vi "Simple Dual Mode Thermometer Facade.vi"(9 "Container State":T3, 10 "Display State In":T2, 11 "Data In":T4) -> (0 "Action":T1, 1 "Display State Out":T2, 3 "Data Out":T4)   [LabVIEW 2023, in "Simple Dual Mode Thermometer XControl.xctl"]
doc: "This VI demonstrates the use of an XControl's Facade VI in implementing a Simple Dual Mode Thermometer. The front panel defines the appearance of the XControl. The block diagram defines the behavior of the XControl."
uses:
  Simple Dual Mode Thermometer XControl.xctl
  Simple Dual Mode Thermometer Data.ctl
  <vilib>/_xctls/Container State.ctl
  Simple Dual Mode Thermometer State.ctl
  <vilib>/_xctls/Action.ctl
  <vilib>/_xctls/XControlSupport.lvlib
panel:
  in  "format string":string="The temperature is %f degrees C or %f degrees F."
  in  "Item Name":string="Display Temperature..."
  in  "Action Name":string="Mode Change"
  in  "Fahrenheit":bool
  in  "Vertical Pointer Slide":dbl(slide) scale=0.0..100.0
  in  "Thermometer":dbl(slide) scale=0.0..100.0
  # "1. Drop the controls that make up the appearance of the XControl here.\n2. Resize the window to fit the controls.\n3. If the XControl is of fixed size,  make the window not resizable from VI Properties->Window Appearance.\n4. If you want the controls to automatically size when the XControl sizes, check  \"Scale all objects on front panel when window resizes\" in File->VI Properties->Window Size page."
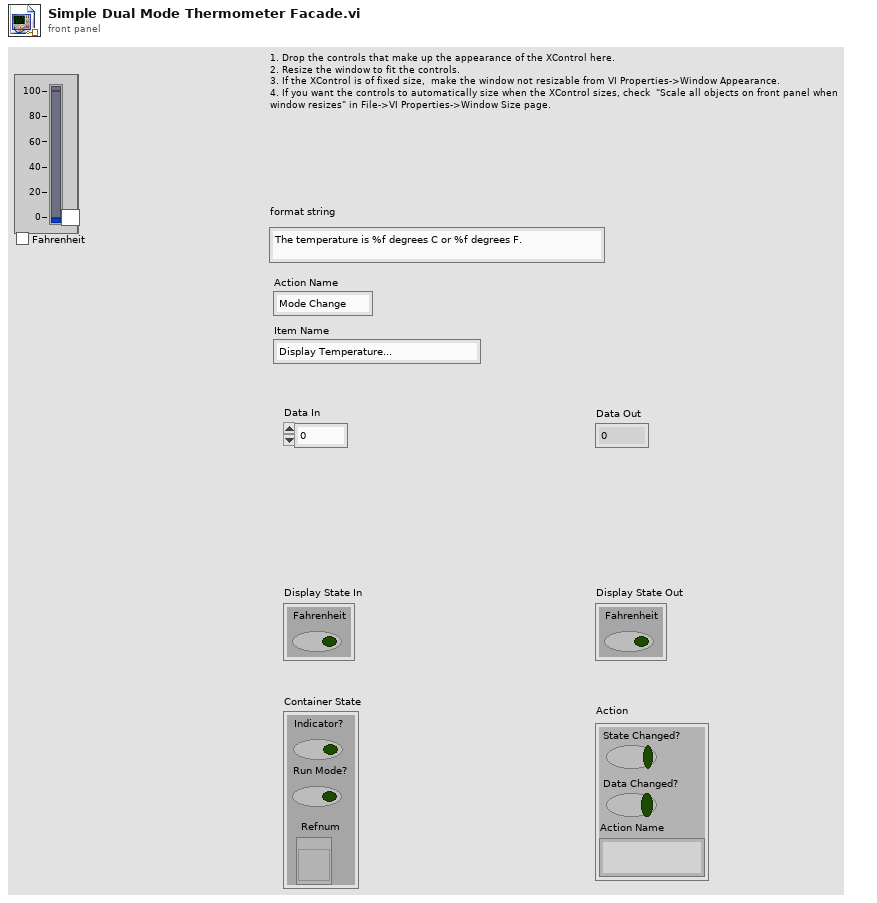
[diagram p1: front panel]
types:
  T1 = typedef "XControlSupport.lvlib/Action.ctl" = cluster{"Data Changed?":bool, "State Changed?":bool, "Action Name":string}
  T2 = typedef "Simple Dual Mode Thermometer XControl.xctl/Simple Dual Mode Thermometer State.ctl" = cluster{"Fahrenheit":bool}
  T3 = typedef "XControlSupport.lvlib/Container State.ctl" = cluster{"Indicator?":bool, "Run Mode?":bool, " Refnum":refnum<vi>}
  T4 = typedef "Simple Dual Mode Thermometer XControl.xctl/Simple Dual Mode Thermometer Data.ctl" = dbl
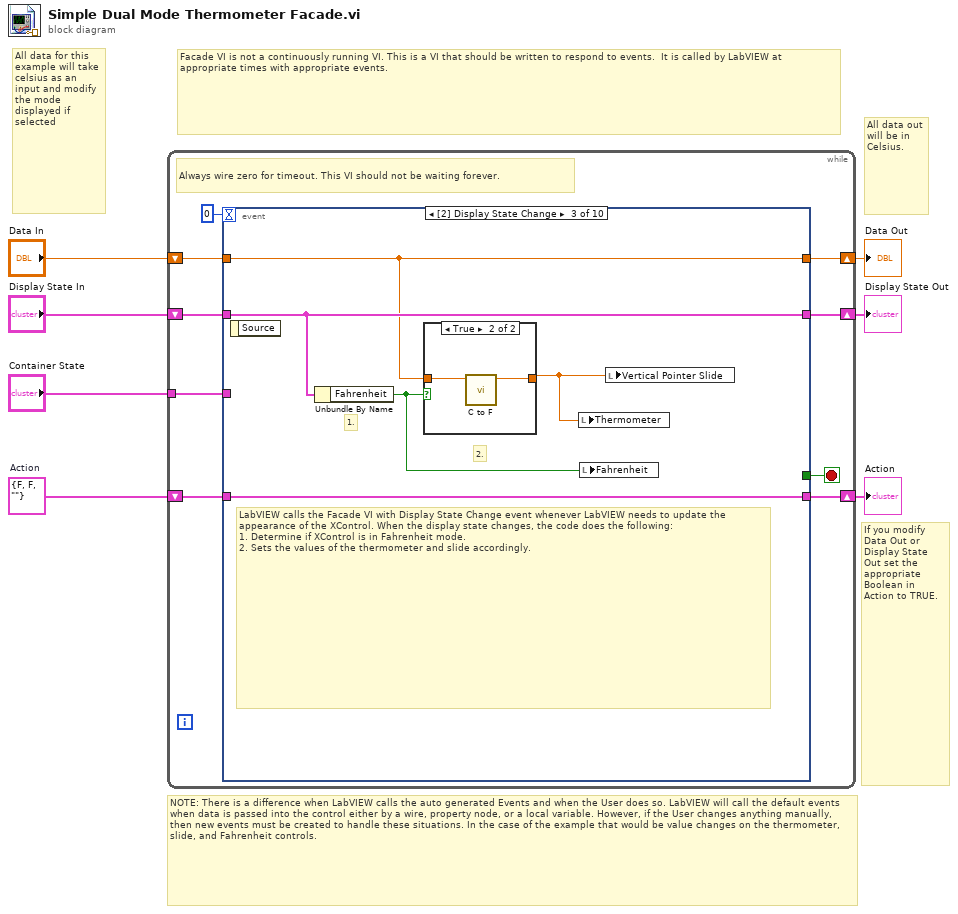
[diagram p0: block diagram]
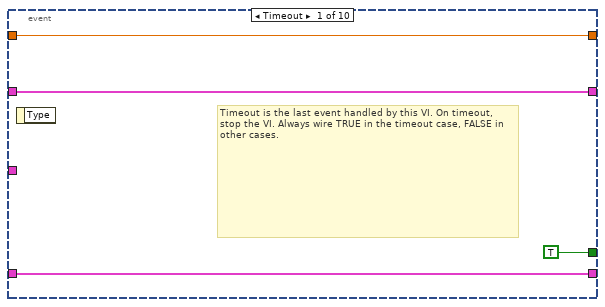
[diagram p2: hidden frame]
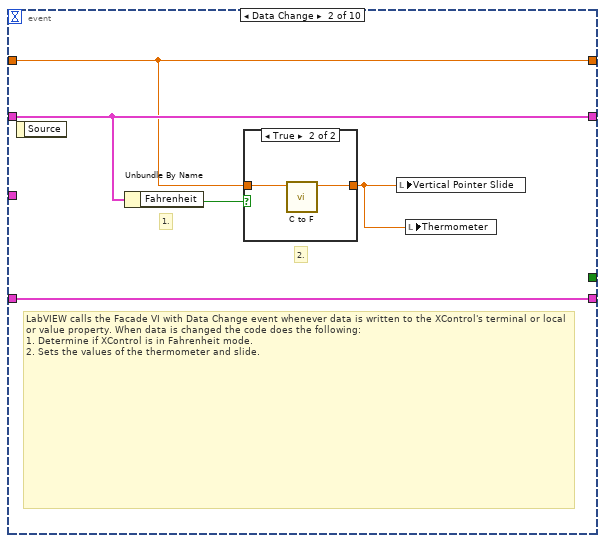
[diagram p3: hidden frame]
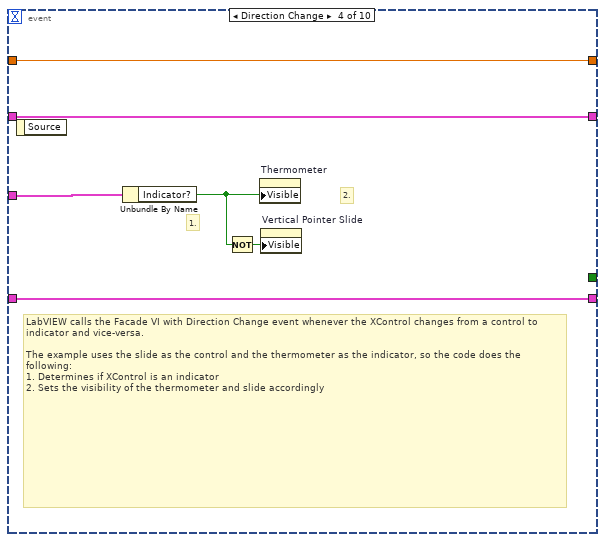
[diagram p6: hidden frame]
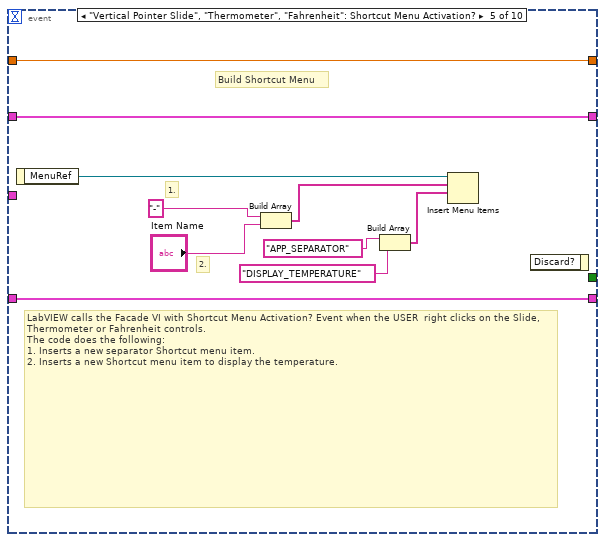
[diagram p7: hidden frame]
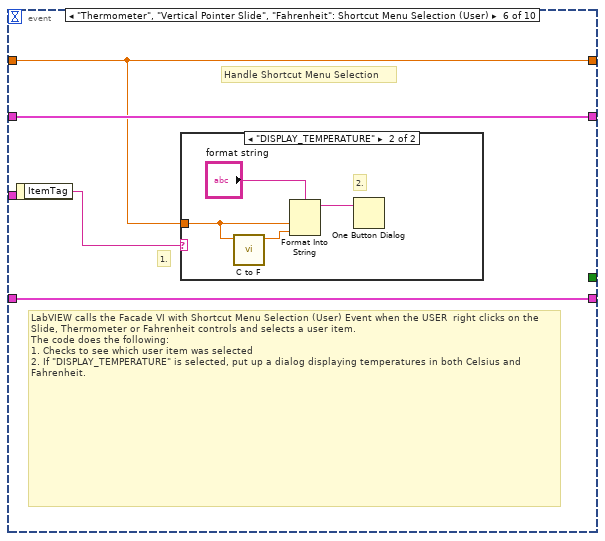
[diagram p8: hidden frame]
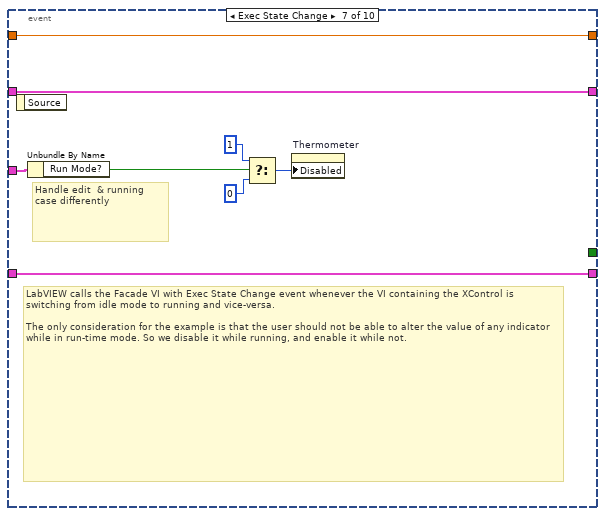
[diagram p10: hidden frame]
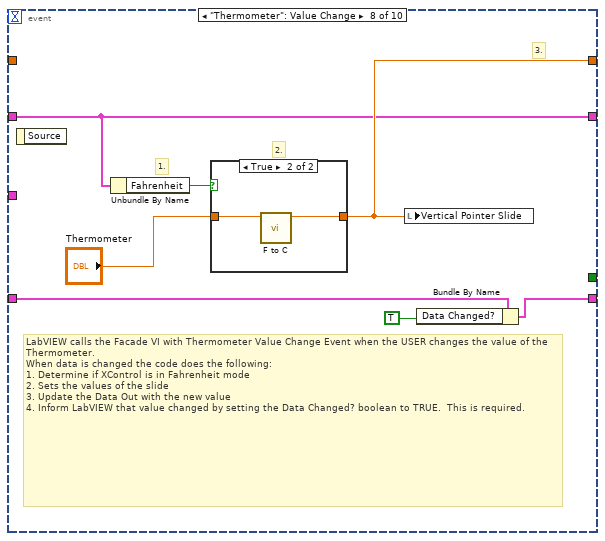
[diagram p11: hidden frame]
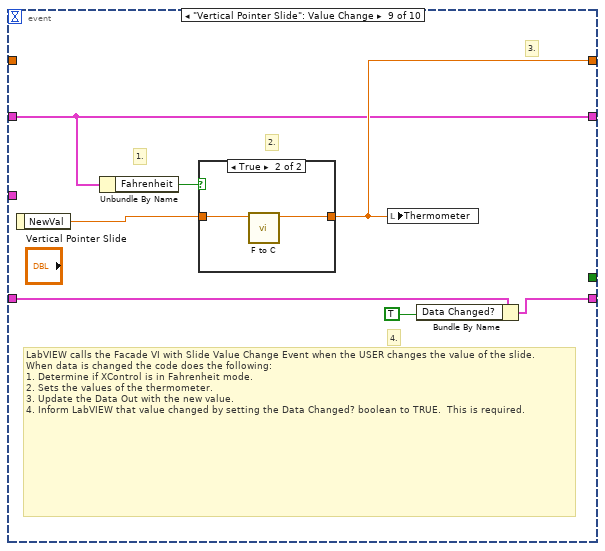
[diagram p13: hidden frame]
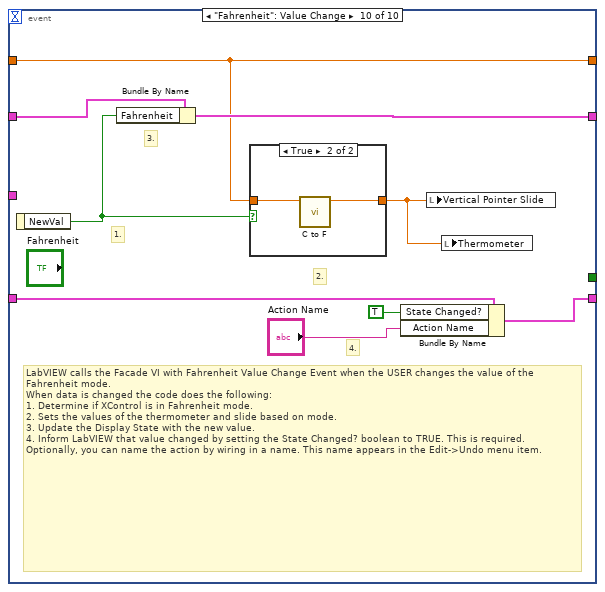
[diagram p15: hidden frame]
diagram:
  w1 = T1 {"Data Changed?"=FALSE, "State Changed?"=FALSE, "Action Name"=""}  # Action
  # "Facade VI is not a continuously running VI. This is a VI that should be written to respond to events.  It is called by LabVIEW at appropriate times with appropriate events."
  # "NOTE: There is a difference when LabVIEW calls the auto generated Events and when the User does so. LabVIEW will call the default events when data is passed into the control either by a wire, property node, or a local variable. However, if the User changes anything manually, then new events must be created to handle these situations. In the case of the example that would be value changes on the thermometer, slide, and Fahrenheit controls."
  # "All data out will be in Celsius."
  # "All data for this example will take celsius as an input and modify the mode displayed if selected"
  # "If you modify Data Out or\nDisplay State Out set the appropriate Boolean in Action to TRUE."
  n1 = while {
    shift-right: [w15] -> w4
    shift-left: "Display State In" -> [w16]
    tunnel: "Container State" -> [w12]
    shift-right: [w10] -> w7
    shift-left: "Data In" -> [w11]
    shift-right: [w8] -> w2
    shift-left: w1 -> [w9]
    stop <- w14 stop-if-true
    # "Always wire zero for timeout. This VI should not be waiting forever."
    n2 = event shown="[2] Display State Change" {
      selector: _ -> [_ _ _ _ _ _ _ _ _ _]
      dyn-events: _ -> [_ _ _ _ _ _ _ _ _ _]
      timeout: 0 -> [_ _ _ _ _ _ _ _ _ _]
      tunnel: w16 -> [w18 w25 w33 w41 w50 w55 w67 w71 w80 w97]
      tunnel: [w18 w25 w33 w41 w50 w55 w67 w71 w80 w96] -> w15
      tunnel: [TRUE _ _ _ _ _ _ _ _ _] -> w14
      tunnel: w12 -> [_ _ _ w42 _ _ w68 _ _ _]
      tunnel: w11 -> [w17 w23 w32 w40 w51 w53 w66 _ _ w95]
      tunnel: [w17 w23 w32 w40 w51 w53 w66 w72 w81 w95] -> w10
      tunnel: [w19 w21 w30 w37 w52 w56 w65 w73 w82 w91] -> w8
      tunnel: w9 -> [w19 w21 w30 w37 w52 w56 w65 w74 w83 w94]
      event Timeout {
        # "Timeout is the last event handled by this VI. On timeout, stop the VI. Always wire TRUE in the timeout case, FALSE in other cases."
        n3 = event-data() -> ()  [unwired: 1 in, 1 out]
      }
      event Data Change {
        # "2."
        # "1."
        # "LabVIEW calls the Facade VI with Data Change event whenever data is written to the XControl's terminal or local or value property. When data is changed the code does the following:\n1. Determine if XControl is in Fahrenheit mode.\n2. Sets the values of the thermometer and slide."
        n4 = event-data() -> ()  [unwired: 1 in, 1 out]
        n5 = Unbundle By Name(w25) -> ("Fahrenheit"=w24:bool)
        n6 = case shown="True" w24 {
          tunnel: w23 -> [w26 w28]
          tunnel: [w26 w27] -> w22
          frame False {
          }
          frame True {
            n7 = call "C to F.vi"("Celsius"=w28) -> ("Fahrenheit"=w27:dbl)  [unwired: 10 in]
          }
        }
        n8 = local write "Vertical Pointer Slide"(w22) -> ()
        n9 = local write "Thermometer"(w22) -> ()
      }
      event Display State Change {
        # "2."
        # "1."
        # "LabVIEW calls the Facade VI with Display State Change event whenever LabVIEW needs to update the appearance of the XControl. When the display state changes, the code does the following:\n1. Determine if XControl is in Fahrenheit mode.\n2. Sets the values of the thermometer and slide accordingly."
        n10 = event-data() -> ()  [unwired: 1 in, 1 out]
        n11 = Unbundle By Name(w33) -> ("Fahrenheit"=w29:bool)
        n12 = case shown="True" w29 {
          tunnel: w32 -> [w34 w36]
          tunnel: [w34 w35] -> w31
          frame False {
          }
          frame True {
            n13 = call "C to F.vi"("Celsius"=w36) -> ("Fahrenheit"=w35:dbl)  [unwired: 10 in]
          }
        }
        n14 = local write "Thermometer"(w31) -> ()
        n15 = local write "Fahrenheit"(w29) -> ()
        n16 = local write "Vertical Pointer Slide"(w31) -> ()
      }
      event Direction Change {
        # "2."
        # "1."
        # "LabVIEW calls the Facade VI with Direction Change event whenever the XControl changes from a control to indicator and vice-versa.\n\nThe example uses the slide as the control and the thermometer as the indicator, so the code does the following: \n1. Determines if XControl is an indicator \n2. Sets the visibility of the thermometer and slide accordingly"
        n17 = event-data() -> ()  [unwired: 1 in, 1 out]
        n18 = Unbundle By Name(w42) -> ("Indicator?"=w38:bool)
        n19 = Not(x=w38) -> (.not. x?=w39:bool)
        n20 = property on="Thermometer" class="Slide (strict)"("Visible"=w38) -> ()  [unwired: 2 in, 2 out]
        n21 = property on="Vertical Pointer Slide" class="Slide (strict)"("Visible"=w39) -> ()  [unwired: 2 in, 2 out]
      }
      event "Vertical Pointer Slide", "Thermometer", "Fahrenheit": Shortcut Menu Activation? {
        # "Build Shortcut Menu"
        # "2."
        # "1."
        # "LabVIEW calls the Facade VI with Shortcut Menu Activation? Event when the USER  right clicks on the Slide, Thermometer or Fahrenheit controls.\nThe code does the following:\n1. Inserts a new separator Shortcut menu item.\n2. Inserts a new Shortcut menu item to display the temperature."
        n22 = event-data() -> ("MenuRef"=w46:refnum<k9>)  [unwired: 1 in]
        n23 = Build Array("-", "Item Name") -> (w47:string[])
        n24 = Build Array("APP_SEPARATOR", "DISPLAY_TEMPERATURE" ("element")) -> (w45:string[])
        n25 = Insert Menu Items(7:w45, 8:w47, 9:w46) -> ()  [unwired: 3 in, 3 out]
        n26 = event-data() -> ()  [unwired: 2 in, 1 out]
      }
      event "Thermometer", "Vertical Pointer Slide", "Fahrenheit": Shortcut Menu Selection (User) {
        # "Handle Shortcut Menu Selection"
        # "1."
        # "LabVIEW calls the Facade VI with Shortcut Menu Selection (User) Event when the USER  right clicks on the Slide, Thermometer or Fahrenheit controls and selects a user item.\nThe code does the following:\n1. Checks to see which user item was selected\n2. If \"DISPLAY_TEMPERATURE\" is selected, put up a dialog displaying temperatures in both Celsius and Fahrenheit."
        n27 = event-data() -> ("ItemTag"=w54:string)  [unwired: 1 in]
        n28 = case shown="\"DISPLAY_TEMPERATURE\"" w54 {
          tunnel: w53 -> [_ w57]
          frame Default {
          }
          frame "DISPLAY_TEMPERATURE" {
            # "2."
            n29 = call "C to F.vi"("Celsius"=w57) -> ("Fahrenheit"=w58:dbl)  [unwired: 10 in]
            n30 = Format Into String(format string="format string", w57, w58) -> (resulting string=w59:string)  [unwired: 2 in, 1 out]
            n31 = One Button Dialog(message=w59) -> ()  [unwired: 1 in, 1 out]
          }
        }
      }
      event Exec State Change {
        # "LabVIEW calls the Facade VI with Exec State Change event whenever the VI containing the XControl is switching from idle mode to running and vice-versa.\n\nThe only consideration for the example is that the user should not be able to alter the value of any indicator while in run-time mode. So we disable it while running, and enable it while not."
        # "Handle edit  & running case differently"
        n32 = event-data() -> ()  [unwired: 1 in, 1 out]
        n33 = Unbundle By Name(w68) -> ("Run Mode?"=w64:bool)
        n34 = Select(t=u8 1 ("Disabled"), s=w64, f=u8 0 ("Disabled")) -> (s? t:f=w61:u8)
        n35 = property on="Thermometer" class="Slide (strict)"("Disabled"=w61) -> ()  [unwired: 2 in, 2 out]
      }
      event "Thermometer": Value Change {
        # "LabVIEW calls the Facade VI with Thermometer Value Change Event when the USER changes the value of the Thermometer.\nWhen data is changed the code does the following:\n1. Determine if XControl is in Fahrenheit mode\n2. Sets the values of the slide\n3. Update the Data Out with the new value\n4. Inform LabVIEW that value changed by setting the Data Changed? boolean to TRUE.  This is required."
        # "3."
        # "2."
        # "1."
        n36 = event-data() -> ()  [unwired: 1 in, 1 out]
        n37 = Unbundle By Name(w71) -> ("Fahrenheit"=w70:bool)
        n38 = case shown="True" w70 {
          tunnel: "Thermometer" -> [w76 w78]
          tunnel: [w76 w77] -> w72
          frame False {
          }
          frame True {
            n39 = call "F to C.vi"("Fahrenheit"=w78) -> ("Celsius"=w77:dbl)  [unwired: 10 in]
          }
        }
        n40 = local write "Vertical Pointer Slide"(w72) -> ()
        n41 = Bundle By Name(cluster=w74, "Data Changed?"=TRUE ("State Changed?")) -> (w73:T1)
      }
      event "Vertical Pointer Slide": Value Change {
        # "4."
        # "3."
        # "2."
        # "1."
        # "LabVIEW calls the Facade VI with Slide Value Change Event when the USER changes the value of the slide.\nWhen data is changed the code does the following:\n1. Determine if XControl is in Fahrenheit mode.\n2. Sets the values of the thermometer.\n3. Update the Data Out with the new value.\n4. Inform LabVIEW that value changed by setting the Data Changed? boolean to TRUE.  This is required."
        n42 = event-data() -> ("NewVal"=w85:dbl)  [unwired: 1 in]
        n43 = Unbundle By Name(w80) -> ("Fahrenheit"=w79:bool)
        n44 = case shown="True" w79 {
          tunnel: w85 -> [w86 w88]
          tunnel: [w86 w87] -> w81
          frame False {
          }
          frame True {
            n45 = call "F to C.vi"("Fahrenheit"=w88) -> ("Celsius"=w87:dbl)  [unwired: 10 in]
          }
        }
        n46 = local write "Thermometer"(w81) -> ()
        n47 = Bundle By Name(cluster=w83, "Data Changed?"=TRUE ("State Changed?")) -> (w82:T1)
      }
      event "Fahrenheit": Value Change {
        # "4."
        # "2."
        # "1."
        # "3."
        # "LabVIEW calls the Facade VI with Fahrenheit Value Change Event when the USER changes the value of the Fahrenheit mode.\nWhen data is changed the code does the following:\n1. Determine if XControl is in Fahrenheit mode.\n2. Sets the values of the thermometer and slide based on mode.\n3. Update the Display State with the new value.\n4. Inform LabVIEW that value changed by setting the State Changed? boolean to TRUE. This is required. Optionally, you can name the action by wiring in a name. This name appears in the Edit->Undo menu item."
        n48 = event-data() -> ("NewVal"=w90:bool)  [unwired: 1 in]
        n49 = Bundle By Name(cluster=w97, "Fahrenheit"=w90) -> (w96:T2)
        n50 = case shown="True" w90 {
          tunnel: w95 -> [w98 w100]
          tunnel: [w98 w99] -> w89
          frame False {
          }
          frame True {
            n51 = call "C to F.vi"("Celsius"=w100) -> ("Fahrenheit"=w99:dbl)  [unwired: 10 in]
          }
        }
        n52 = Bundle By Name(cluster=w94, "State Changed?"=TRUE, "Action Name"="Action Name") -> (w91:T1)
        n53 = local write "Vertical Pointer Slide"(w89) -> ()
        n54 = local write "Thermometer"(w89) -> ()
      }
    }
  }
  "Display State Out" <- w4
  "Data Out" <- w7
  "Action" <- w2
